vi "Synchronization State Machine.vi"(6 "sync input sample valid":bool=TRUE, 7 "consecutive peaks for preamble detection":u8, 8 "rearm packet detection":bool=TRUE, 9 "packet start":bool=TRUE, 10 "number of consecutive peaks valid":bool=TRUE, 11 "consecutive peak count":u8) -> (1 "reset peak count":bool=TRUE, 2 "packet detected":bool=TRUE)   [LabVIEW 2020]
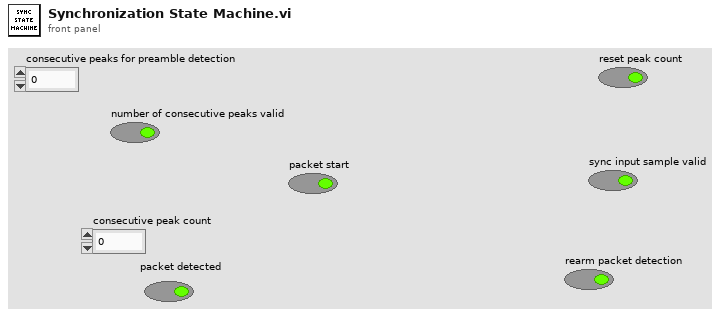
[diagram p1: front panel]
types:
  T1 = enum16{"\"detect preamble candidate\"", "\"detect full preamble\"", "\"wait for possible extra correlation peak\"", "\"sync not armed\""}
  T2 = cluster{"EIFS":u32, "ACK timeout":u32, "CTS timeout":u32, "aRxPHYStartDelay":u32, "Frame control field length":u16, "Duration/ID field length":u16, "aSlotTime":u32, "aSIFSTime":u32, "PIFS":u32, "DIFS":u32, "Address field length":u16, "Sequence control field length":u16, "QoS control field length":u16, "HT control field length":u16, "FCS field length":u16, "MPDU delimiter length":u16, "MPDU delimiter signature":u16, "Max MPDU buffer length":u16, "timestamp steps / mks":u32, "L-STF periods / L-STF":u8, "sample / L-STF period":u8, "T_SIGNAL":u16, "N_tail":u16, "N_service":u16, "N_ES":u16, "N_SS":u16, "m_STBC":u16, "T_VHTSIGB":u16, "T_VHTPREAMBLE":u16, "T_VHTSIGA":u16, "T_LSIG":u16, "T_LEGPREAMBLE":u16, "NOFDM_VHTSIGB":u16, "T_SYM":u16, "T_SYML":u16, "NOFDM_PREAMBLE":u16, "NOFDM_SIGNAL":u16, "T_PREAMBLE":u16, "NOFDM_LEGPREAMBLE":u16, "NOFDM_VHTPREAMBLE":u16, "NOFDM_VHTSIGA":u16, "NOFDM_LSIG":u16, "NOFDM_VHTPREAMBLE 2":u16, "NOFDM_LSIG 2":u16}
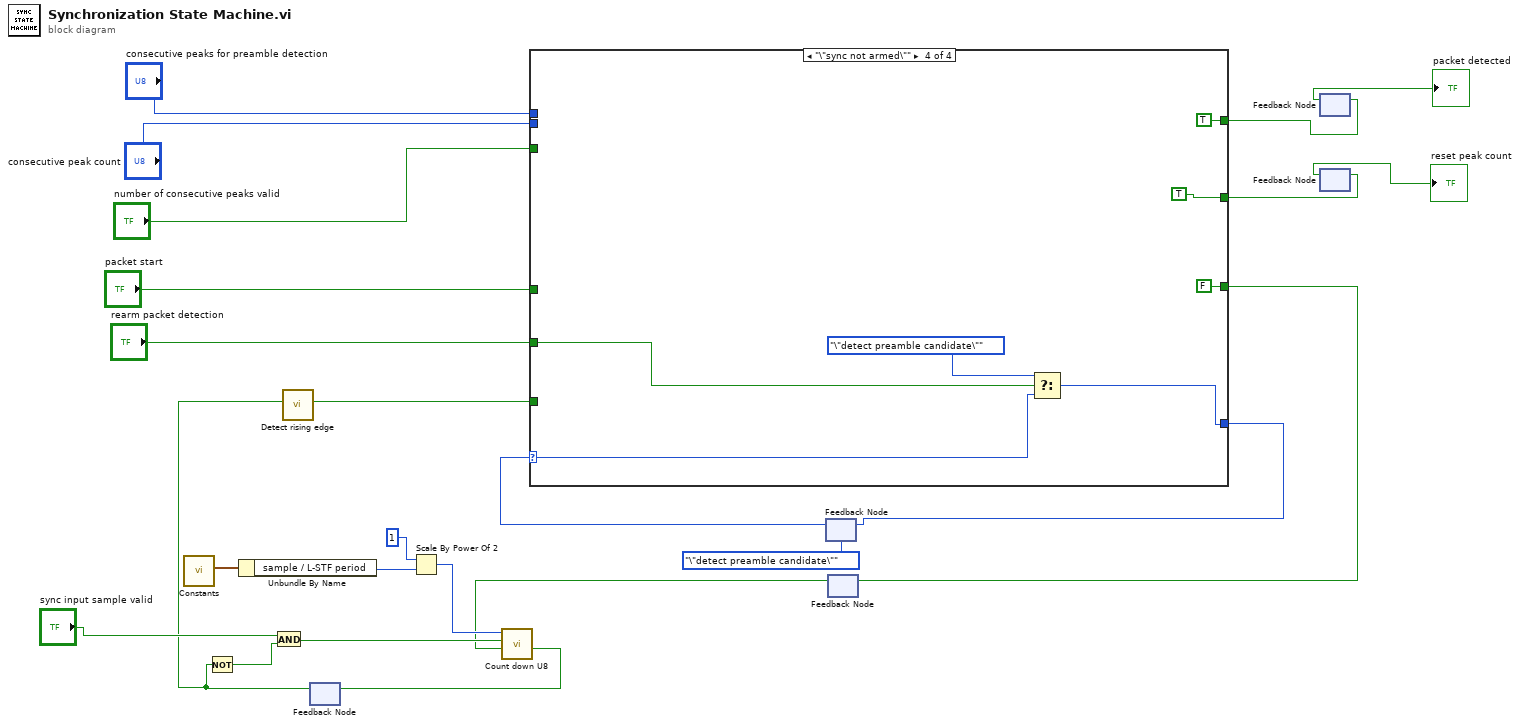
[diagram p0: block diagram]
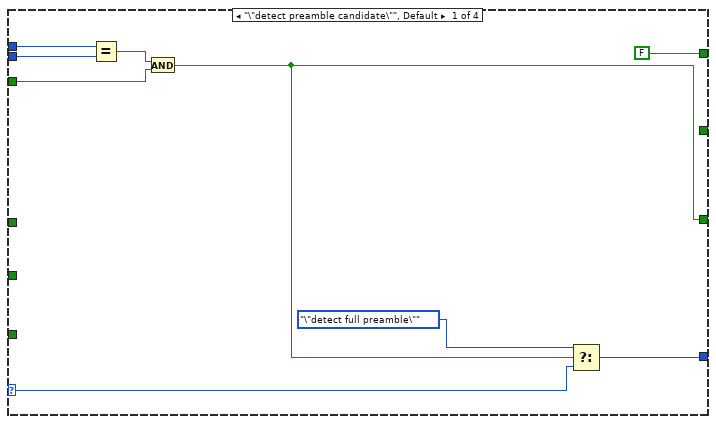
[diagram p2: hidden frame]
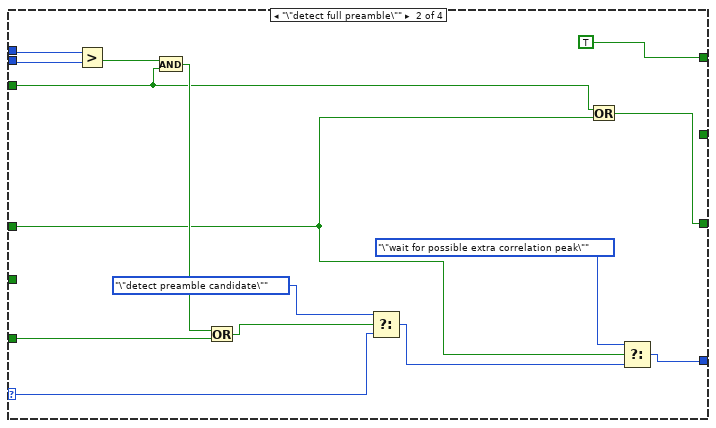
[diagram p3: hidden frame]
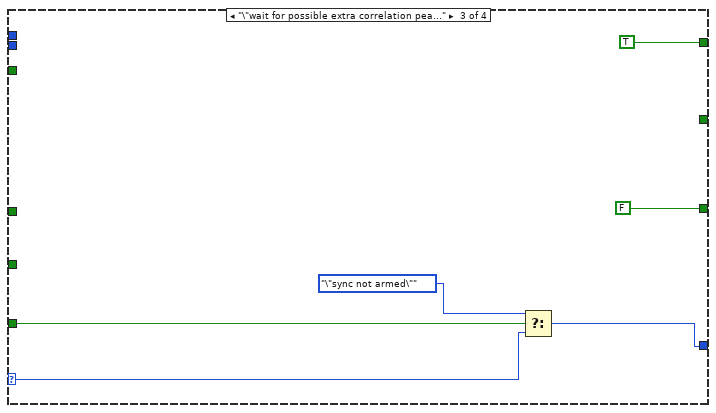
[diagram p4: hidden frame]
diagram:
  n1 = call "Constants.vi"() -> ("output cluster"=w9:T2)  [unwired: 11 in]
  n2 = Unbundle By Name(w9) -> ("sample / L-STF period"=w7:u8)
  n3 = feedback #1() -> (w10:bool)  [unwired: 1 in]
  n4 = Not(x=w10) -> (.not. x?=w13:bool)
  n5 = And(x="sync input sample valid", y=w13) -> (x .and. y?=w11:bool)
  n6 = call "Detect rising edge.vi"("signal"=w10) -> ("edge detected"=w15:bool)  [unwired: 10 in]
  n7 = Scale By Power Of 2(n=i16 1, x=w7) -> (x*2^n=w6:u8)
  n8 = feedback #2(T1."\"detect preamble candidate\"") -> (w23:T1)
  n9 = case shown="\"\\\"sync not armed\\\"\"" w23 {
    selector: w23 -> [w27 w37 w52 w60]
    tunnel: "consecutive peaks for preamble detection" -> [w33 w47 _ _]
    tunnel: "consecutive peak count" -> [w32 w46 _ _]
    tunnel: "number of consecutive peaks valid" -> [w30 w34 _ _]
    tunnel: [w29 w42 w51 w55] -> w19
    tunnel: [FALSE TRUE TRUE TRUE] -> w17
    tunnel: w15 -> [_ w40 w54 _]
    tunnel: [w25 w43 FALSE FALSE] -> w4
    tunnel: "rearm packet detection" -> [_ _ _ w59]
    tunnel: [_ _ _ TRUE] -> w2
    tunnel: "packet start" -> [_ w35 _ _]
    frame "\"detect preamble candidate\"", Default {
      n10 = Equal?(x=w33, y=w32) -> (x = y?=w31:bool)
      n11 = And(x=w31, y=w30) -> (x .and. y?=w25:bool)
      n12 = Select(t=T1."\"detect full preamble\"", s=w25, f=w27) -> (s? t:f=w29:T1)
    }
    frame "\"detect full preamble\"" {
      n13 = Greater?(x=w47, y=w46) -> (0:w45:bool)
      n14 = And(x=w45, y=w34) -> (x .and. y?=w39:bool)
      n15 = Or(x=w39, y=w40) -> (x .or. y?=w38:bool)
      n16 = Select(t=T1."\"detect preamble candidate\"", s=w38, f=w37) -> (s? t:f=w41:T1)
      n17 = Or(x=w34, y=w35) -> (x .or. y?=w43:bool)
      n18 = Select(t=T1."\"wait for possible extra correlation peak\"", s=w35, f=w41) -> (s? t:f=w42:T1)
    }
    frame "\"wait for possible extra correlation peak\"" {
      n19 = Select(t=T1."\"sync not armed\"", s=w54, f=w52) -> (s? t:f=w51:T1)
    }
    frame "\"sync not armed\"" {
      n20 = Select(t=T1."\"detect preamble candidate\"", s=w59, f=w60) -> (s? t:f=w55:T1)
    }
  }
  n21 = feedback-in #2(w19) -> ()
  n22 = feedback #3() -> (w5:bool)  [unwired: 1 in]
  n23 = call "Count down U8.vi"("load"=w5, "decrement"=w11, "count in"=w6) -> ("terminal count"=w12:bool)  [unwired: 7 in, 1 out]
  n24 = feedback-in #1(w12) -> ()
  n25 = feedback-in #3(w4) -> ()
  n26 = feedback #4() -> (→"packet detected":bool)  [unwired: 1 in]
  n27 = feedback-in #4(w17) -> ()
  n28 = feedback #5() -> (→"reset peak count":bool)  [unwired: 1 in]
  n29 = feedback-in #5(w2) -> ()
